vi "Create_BSA_optim_table.vi"(4 "No of samples+extra":i32, 7 "BSA No":enum16{"BSA 1", "BSA 2"}(ring)) -> (2 "BSA results":string[](array[string]))   [LabVIEW 2010]
uses:
  Globals/Dynamic_call_global.ph.vi
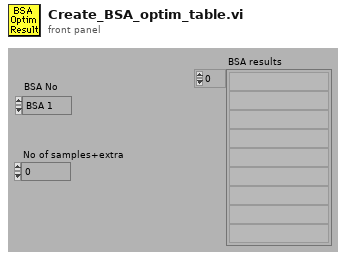
[diagram p1: front panel]
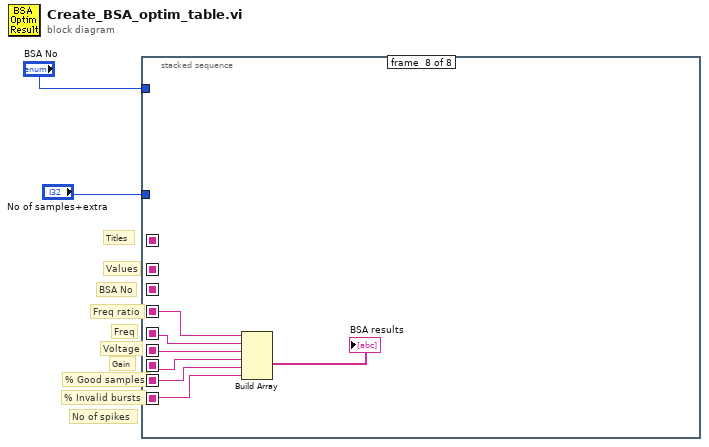
[diagram p0: block diagram]
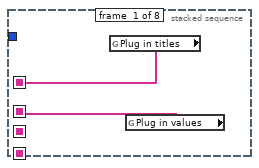
[diagram p2: hidden frame]
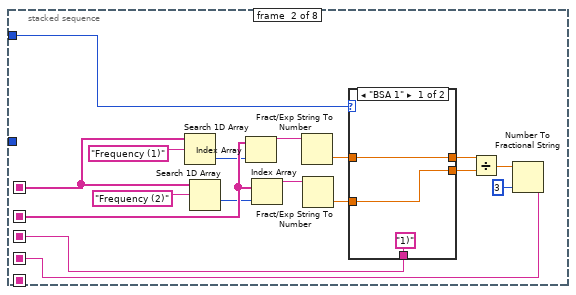
[diagram p3: hidden frame]
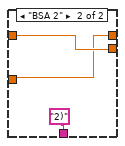
[diagram p4: hidden frame]
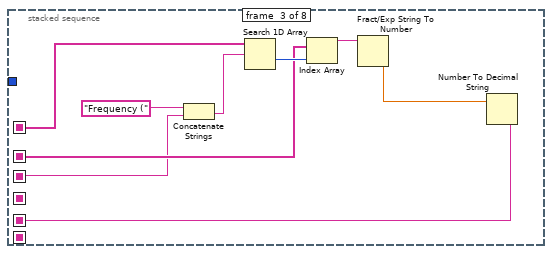
[diagram p5: hidden frame]
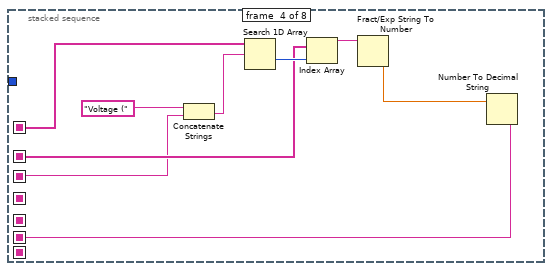
[diagram p6: hidden frame]
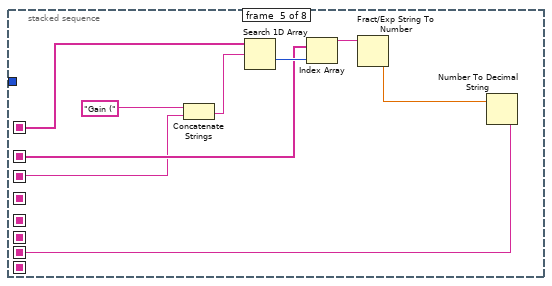
[diagram p7: hidden frame]
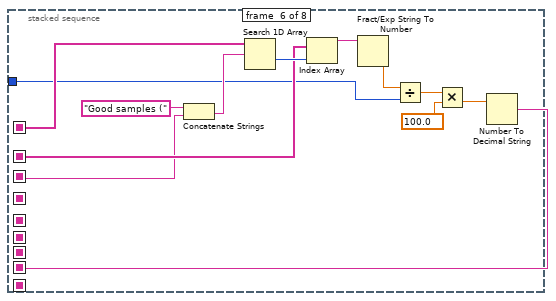
[diagram p8: hidden frame]
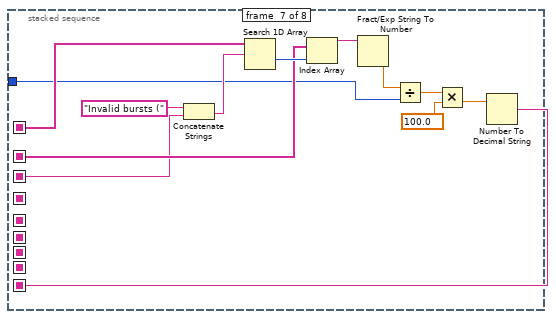
[diagram p9: hidden frame]
diagram:
  # "Gain"
  # "Voltage"
  # "Freq"
  # "No of spikes"
  # "% Invalid bursts"
  # "% Good samples"
  # "BSA No"
  # "Freq ratio"
  # "Values"
  # "Titles"
  n1 = stacked-sequence {
    seq-local: [w4 _ _ _ _ _ _ _] -> [_ w20 w34 w43 w52 w65 w78 _]
    seq-local: [w3 _ _ _ _ _ _ _] -> [_ w18 w33 w42 w51 w64 w77 _]
    seq-local: [_ w12 _ _ _ _ _ _] -> [_ _ _ _ _ _ _ w81]
    seq-local: [_ w10 _ _ _ _ _ _] -> [_ _ w31 w40 w49 w62 w75 _]
    seq-local: [_ _ _ _ _ w56 _ _] -> [_ _ _ _ _ _ _ w86]
    seq-local: [_ _ _ _ _ _ w69 _] -> [_ _ _ _ _ _ _ w85]
    seq-local: [_ _ w28 _ _ _ _ _] -> [_ _ _ _ _ _ _ w82]
    seq-local: [_ _ _ w37 _ _ _ _] -> [_ _ _ _ _ _ _ w83]
    seq-local: [_ _ _ _ w46 _ _ _] -> [_ _ _ _ _ _ _ w84]
    tunnel: "No of samples+extra" -> [_ _ _ _ _ w55 w68 _]
    tunnel: "BSA No" -> [_ w9 _ _ _ _ _ _]
    frame #0 {
      n2 = global read "Dynamic_call_global.ph.vi" "Plug in titles"() -> (w4:string[])
      n3 = global read "Dynamic_call_global.ph.vi" "Plug in values"() -> (w3:string[])
    }
    frame #1 {
      n4 = Search 1D Array(1D array=w20, element="Frequency (1)") -> (index of element=w16:i32)  [unwired: 1 out]
      n5 = Search 1D Array(1D array=w20, element="Frequency (2)") -> (index of element=w17:i32)  [unwired: 1 out]
      n6 = Index Array(array=w18, index=w16) -> (element=w15:string)
      n7 = Index Array(array=w18, index=w17) -> (element=w14:string)
      n8 = Fract/Exp String To Number(string=w15) -> (number=w7:dbl)  [unwired: 4 out]
      n9 = Fract/Exp String To Number(string=w14) -> (number=w6:dbl)  [unwired: 4 out]
      n10 = case shown="\"BSA 1\"" w9 {
        tunnel: ["1)" "2)"] -> w10
        tunnel: [w23 w26] -> w8
        tunnel: w7 -> [w23 w27]
        tunnel: w6 -> [w22 w26]
        tunnel: [w22 w27] -> w5
        frame "BSA 1" {
        }
        frame "BSA 2" {
        }
      }
      n11 = Divide(x=w8, y=w5) -> (x/y=w13:dbl)
      n12 = Number To Fractional String(number=w13, precision (6)=i16 3) -> (F-format string=w12:string)  [unwired: 2 out]
    }
    frame #2 {
      n13 = Concatenate Strings("Frequency (", w31) -> (w30:string)
      n14 = Search 1D Array(1D array=w34, element=w30) -> (index of element=w36:i32)  [unwired: 1 out]
      n15 = Index Array(array=w33, index=w36) -> (element=w35:string)
      n16 = Fract/Exp String To Number(string=w35) -> (number=w29:dbl)  [unwired: 4 out]
      n17 = Number To Decimal String(number=w29) -> (decimal integer string=w28:string)  [unwired: 1 out]
    }
    frame #3 {
      n18 = Concatenate Strings("Voltage (", w40) -> (w39:string)
      n19 = Search 1D Array(1D array=w43, element=w39) -> (index of element=w45:i32)  [unwired: 1 out]
      n20 = Index Array(array=w42, index=w45) -> (element=w44:string)
      n21 = Fract/Exp String To Number(string=w44) -> (number=w38:dbl)  [unwired: 4 out]
      n22 = Number To Decimal String(number=w38) -> (decimal integer string=w37:string)  [unwired: 1 out]
    }
    frame #4 {
      n23 = Concatenate Strings("Gain (", w49) -> (w48:string)
      n24 = Search 1D Array(1D array=w52, element=w48) -> (index of element=w54:i32)  [unwired: 1 out]
      n25 = Index Array(array=w51, index=w54) -> (element=w53:string)
      n26 = Fract/Exp String To Number(string=w53) -> (number=w47:dbl)  [unwired: 4 out]
      n27 = Number To Decimal String(number=w47) -> (decimal integer string=w46:string)  [unwired: 1 out]
    }
    frame #5 {
      n28 = Concatenate Strings("Good samples (", w62) -> (w61:string)
      n29 = Search 1D Array(1D array=w65, element=w61) -> (index of element=w67:i32)  [unwired: 1 out]
      n30 = Index Array(array=w64, index=w67) -> (element=w66:string)
      n31 = Fract/Exp String To Number(string=w66) -> (number=w60:dbl)  [unwired: 4 out]
      n32 = Divide(x=w60, y=w55) -> (x/y=w58:dbl)
      n33 = Multiply(x=w58, y=100.0) -> (x*y=w57:dbl)
      n34 = Number To Decimal String(number=w57) -> (decimal integer string=w56:string)  [unwired: 1 out]
    }
    frame #6 {
      n35 = Concatenate Strings("Invalid bursts (", w75) -> (w74:string)
      n36 = Search 1D Array(1D array=w78, element=w74) -> (index of element=w80:i32)  [unwired: 1 out]
      n37 = Index Array(array=w77, index=w80) -> (element=w79:string)
      n38 = Fract/Exp String To Number(string=w79) -> (number=w73:dbl)  [unwired: 4 out]
      n39 = Divide(x=w73, y=w68) -> (x/y=w71:dbl)
      n40 = Multiply(x=w71, y=100.0) -> (x*y=w70:dbl)
      n41 = Number To Decimal String(number=w70) -> (decimal integer string=w69:string)  [unwired: 1 out]
    }
    frame #7 {
      n42 = Build Array(w81, w82, w83, w84, w86, w85) -> (→"BSA results":string[])
    }
  }
